vi "Hex to Float.vi"(11 "read buffer in":string="\u0002\u0003\u0004_ÿ¼ê\u001aX") -> (2 "Floating Point":sgl=-0.028610228, 3 "read buffer out":string="_ÿ¼ê")   [LabVIEW 2016]
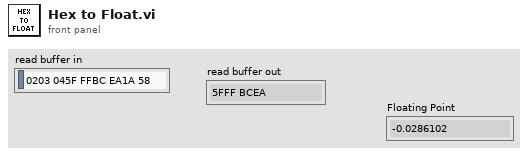
[diagram p1: front panel]
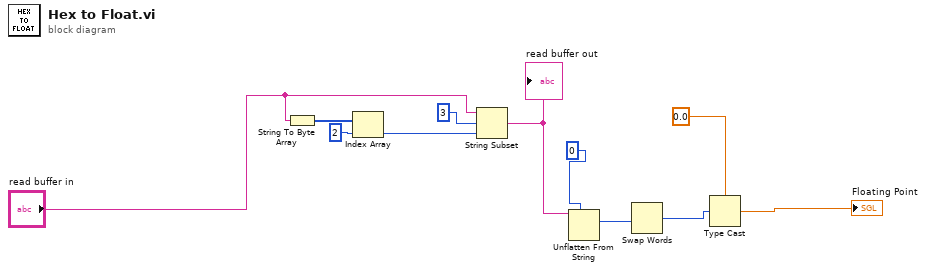
[diagram p0: block diagram]
diagram:
  n1 = String To Byte Array(string="read buffer in") -> (unsigned byte array=w8:u8[])
  n2 = Index Array(array=w8, index=2) -> (element=w10:u8)
  n3 = String Subset(string="read buffer in", offset (0)=3, length (rest)=w10) -> (substring=w6:string)
  "read buffer out" <- w6
  n4 = Unflatten From String(type=0, binary string=w6) -> (value=w2:i32)  [unwired: 3 in, 2 out]
  n5 = Swap Words(1:w2) -> (0:w4:i32)
  n6 = Type Cast(type=sgl 0.0, x=w4) -> (*(type *) &x=→"Floating Point":sgl)
